vi "GL CheckForMotion.vi"(8 "error in":errorcluster, 10 "Axis":T1 items=["Axis 1", "Axis 2", "Axis 3", "Axis 4", "Axis 5", "Axis 6", "Axis 7", "Axis 8"], 11 "Refnum in":refnum<k7>) -> (0 "error out":errorcluster, 2 "Axis out":T1 items=["Axis 1", "Axis 2", "Axis 3", "Axis 4", "Axis 5", "Axis 6", "Axis 7", "Axis 8"], 3 "Refnum out":refnum<k7>)   [LabVIEW 2022 SP3]
uses:
  GL Axis Control.ctl
  Command Menu.ctl
panel:
  out "Stop State":string
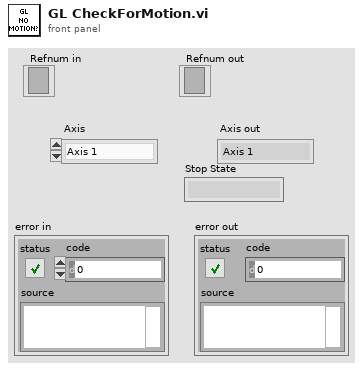
[diagram p1: front panel]
types:
  T1 = typedef "GL Axis Control.ctl" = u16
  T2 = typedef "Command Menu.ctl" = enum16{"CommandPassThrough", "Abort Motion", "Define Pos", "Velocity", "Acceleration", "Deceleration", "Position Rel", "Postion Abs", "Begin Move", "After Move", "Home", "KI", "KD", "KP", "IL", "Config I/O", "Set Bit", "Clear Bit", "Motor Off", "Moto On", "Status", "Execute", "Halt Execute", "HX Status", "Tell Velocity", "Check Motion", "BreakPoint", "Tell Position", "Current Code Line", "Tell Switches", "OC Force On", "OC Off", "Pos Soft Limit", "Rev Soft Limit"}
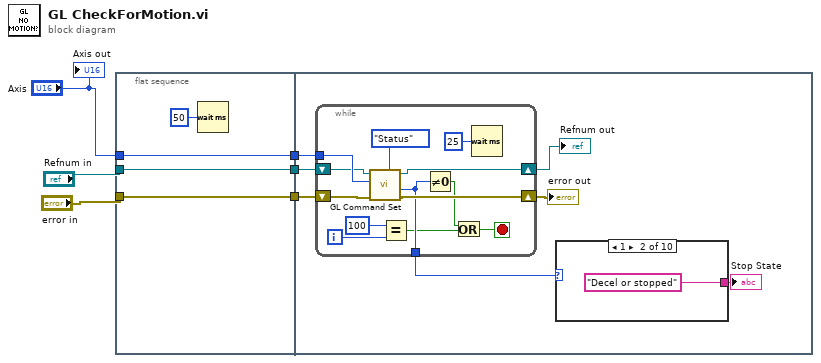
[diagram p0: block diagram]
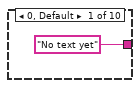
[diagram p2: hidden frame]
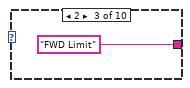
[diagram p3: hidden frame]
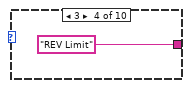
[diagram p4: hidden frame]
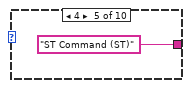
[diagram p5: hidden frame]
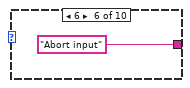
[diagram p6: hidden frame]
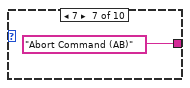
[diagram p7: hidden frame]
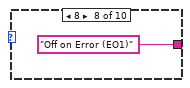
[diagram p8: hidden frame]
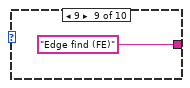
[diagram p9: hidden frame]
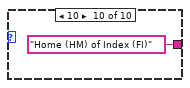
[diagram p10: hidden frame]
diagram:
  n1 = flat-sequence {
    tunnel: "Axis" -> [w8]
    tunnel: "Refnum in" -> [w9]
    tunnel: "error in" -> [w10]
    tunnel: [w10] -> w3
    tunnel: [w9] -> w2
    tunnel: [w8] -> w1
    tunnel: w3 -> [w16]
    tunnel: w2 -> [w15]
    tunnel: w1 -> [w13]
    frame #0 {
      n2 = Wait (ms)(milliseconds to wait=u32 50) -> ()  [unwired: 1 out]
    }
    frame #1 {
      n3 = while {
        shift-right: [w35] -> w17
        shift-left: w16 -> [w34]
        shift-right: [w36] -> w14
        shift-left: w15 -> [w37]
        tunnel: w13 -> [w38]
        tunnel: [w33] -> w12
        i -> [w32]
        stop <- w28 stop-if-true
        n4 = call "GL Command Set.vi"("Command"=Command_Menu."Status", "error in (no error)"=w34, "Axis"=w38, "Galil.IGalil"=w37) -> ("error out"=w35:errorcluster, "Response#"=w33:i32, "ref out"=w36:refnum<k7>)  [unwired: 3 in, 2 out]
        n5 = Equal?(x=100, y=w32) -> (x = y?=w30:bool)
        n6 = Not Equal To 0?(x=w33) -> (x != 0?=w29:bool)
        n7 = Or(x=w29, y=w30) -> (x .or. y?=w28:bool)
        n8 = Wait (ms)(milliseconds to wait=u32 25) -> ()  [unwired: 1 out]
      }
      "error out" <- w17
      "Refnum out" <- w14
      n9 = case shown="1" w12 {
        tunnel: ["No text yet" "Decel or stopped" "FWD Limit" "REV Limit" "ST Command (ST)" "Abort input" "Abort Command (AB)" "Off on Error (EO1)" "Edge find (FE)" "Home (HM) of Index (FI)"] -> w11
        frame 0, Default {
        }
        frame 1 {
        }
        frame 2 {
        }
        frame 3 {
        }
        frame 4 {
        }
        frame 6 {
        }
        frame 7 {
        }
        frame 8 {
        }
        frame 9 {
        }
        frame 10 {
        }
      }
      "Stop State" <- w11
    }
  }
  "Axis out" <- "Axis"
